vi "RSZVB Set Linearity Deviation State.vi"(8 "error in (no error)":errorcluster {"code" format="%.0x"}, 9 "State (2)":i32(ring)=2 items=["Off", "On", "Tracking"], 10 "Channel (1)":i32=1, 11 "VISA session":refnum<visa-resource-name>) -> (0 "error out":errorcluster {"code" format="%.0x"}, 3 "dup VISA session":refnum<visa-resource-name>)   [LabVIEW 2011]
doc: "This VI applies /discards the correction factors or re-calculates them for each trace (Tracking). \n\nRemote-control command(s):\nCALCulate<Chn>:LDEViation:MODE ON | OFF | TRACking"
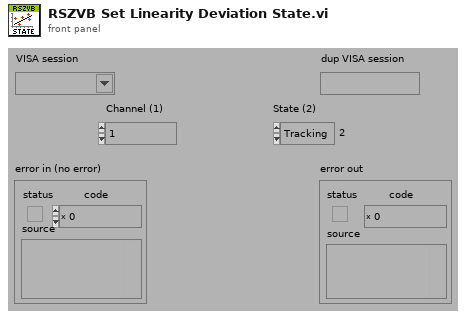
[diagram p1: front panel]
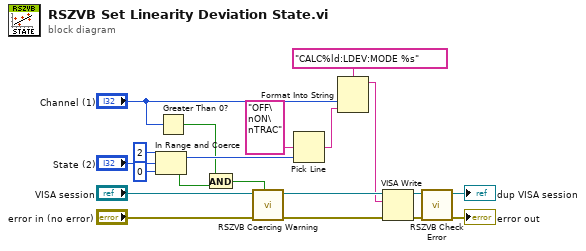
[diagram p0: block diagram]
diagram:
  n1 = In Range and Coerce(upper limit=2, x="State (2)", lower limit=0) -> (coerced(x)=w3:i32, In Range?=w4:bool)
  n2 = Greater Than 0?(x="Channel (1)") -> (x > 0?=w1:bool)
  n3 = And(x=w1, y=w4) -> (x .and. y?=w5:bool)
  n4 = call "RSZVB Coercing Warning.vi"("In Range?"=w5, "error in (no error)"="error in (no error)", "VISA session"="VISA session") -> ("error out"=w16:errorcluster, "dup VISA session"=w15:refnum<visa-resource-name>)  [unwired: 7 in]
  n5 = Pick Line(multi-line string="OFF\nON\nTRAC", line index=w3) -> (output string=w10:string)  [unwired: 1 in]
  n6 = Format Into String(format string="CALC%ld:LDEV:MODE %s", "Channel (1)", w10) -> (resulting string=w9:string)  [unwired: 2 in, 1 out]
  n7 = VISA Write(VISA resource name=w15, write buffer=w9, error in (no error)=w16) -> (VISA resource name out=w13:refnum<visa-resource-name>, error out=w14:errorcluster)  [unwired: 1 out]
  n8 = call "RSZVB Check Error.vi"("error in (no error)"=w14, "VISA session"=w13) -> ("error out"=→"error out":errorcluster, "dup VISA session"=→"dup VISA session":refnum<visa-resource-name>)  [unwired: 8 in]
